vi "Rename Node.vi"(8 "error in (no error)":errorcluster, 9 "New Name":string, 10 "Old Name":string, 11 "FSM.Edge in":refnum<class "FSM.Edge.lvclass">) -> (0 "error out":errorcluster, 3 "FSM.Edge out":refnum<class "FSM.Edge.lvclass">)   [LabVIEW 2015, in "FSM.Edge.lvclass"]
uses:
  FSM.Edge.lvclass
  FSM.Edge.lvclass/FSM.Edge.ctl
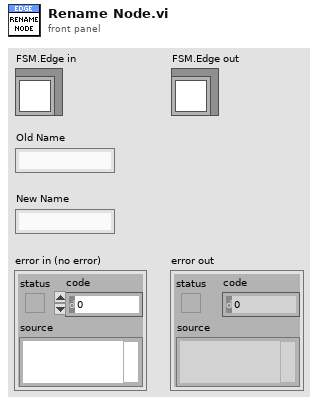
[diagram p1: front panel]
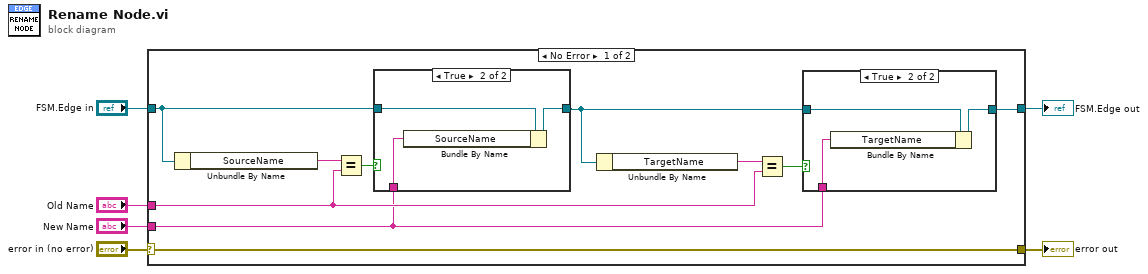
[diagram p0: block diagram]
diagram:
  n1 = case shown="No Error" "error in (no error)" {
    selector: "error in (no error)" -> [w16 w26]
    tunnel: [w16 w26] -> w5
    tunnel: [w10 w25] -> w3
    tunnel: "FSM.Edge in" -> [w13 w25]
    tunnel: "Old Name" -> [w8 _]
    tunnel: "New Name" -> [w7 _]
    frame No Error {
      n2 = Unbundle By Name(w13) -> ("SourceName"=w14:string)
      n3 = Equal?(x=w14, y=w8) -> (x = y?=w15:bool)
      n4 = case shown="True" w15 {
        tunnel: w13 -> [w21 w24]
        tunnel: [w21 w23] -> w9
        tunnel: w7 -> [_ w22]
        frame False {
        }
        frame True {
          n5 = Bundle By Name(cluster=w24, "SourceName"=w22) -> (w23:refnum<class "FSM.Edge.lvclass">)
        }
      }
      n6 = Unbundle By Name(w9) -> ("TargetName"=w11:string)
      n7 = Equal?(x=w11, y=w8) -> (x = y?=w12:bool)
      n8 = case shown="True" w12 {
        tunnel: w9 -> [w17 w20]
        tunnel: [w17 w19] -> w10
        tunnel: w7 -> [_ w18]
        frame False {
        }
        frame True {
          n9 = Bundle By Name(cluster=w20, "TargetName"=w18) -> (w19:refnum<class "FSM.Edge.lvclass">)
        }
      }
    }
    frame Error {
    }
  }
  "error out" <- w5
  "FSM.Edge out" <- w3
